vi "DSF.Engine.Interface.RT FIFO.Create.vi"   [LabVIEW 2017, in "Data Sharing Framework Engine.lvlib" / "DSF.Engine.Interface.lvclass"]
uses:
  DSF.Engine.Interface.lvclass
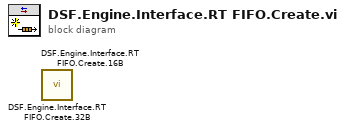
[diagram p0: block diagram]
diagram:
  n1 = call "DSF.Engine.Interface.RT FIFO.Create.32B.vi"() -> ()  [unwired: 10 in, 2 out]
  n2 = call "DSF.Engine.Interface.RT FIFO.Create.16B.vi"() -> ()  [unwired: 10 in, 2 out]
